vi "TCPIP_AcquisitionChA.vi"() -> ()   [LabVIEW 2018]
panel:
  out "error out 5":errorcluster
  out "error out":errorcluster
  in  "stop":bool
  out "error out 4":errorcluster
  out "error out 3":errorcluster
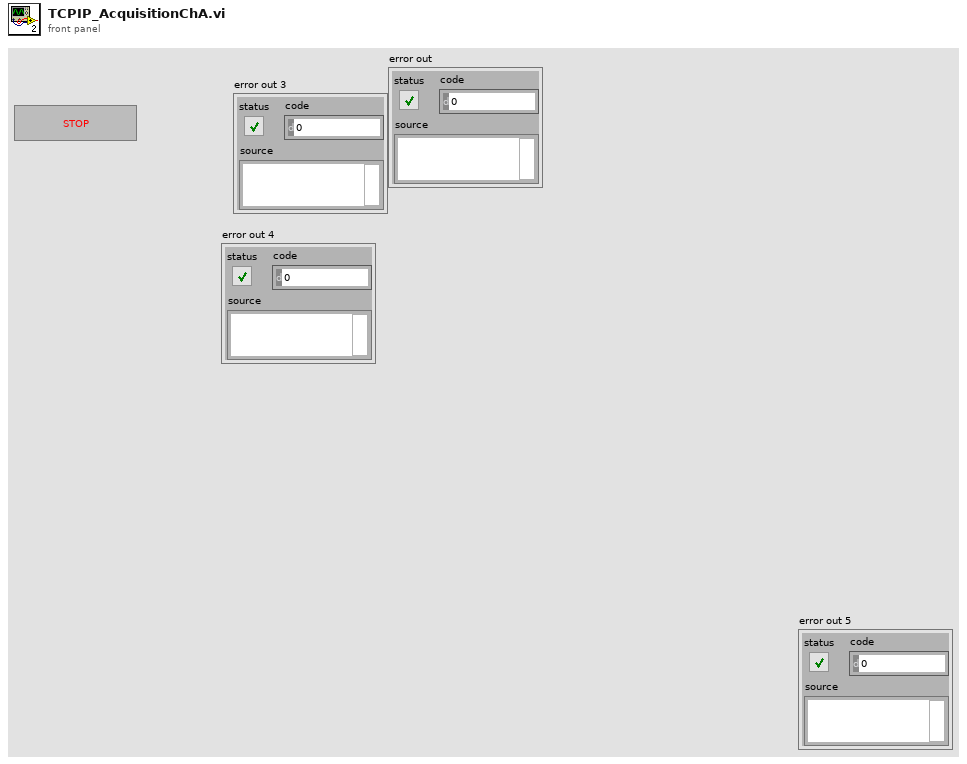
[diagram p1: front panel]
types:
  T1 = cluster{"ID":u32, "Address":string, "Service Name 1":string, "Service Name 2":string, "queue TX":refnum<queue>, "queue RX":refnum<queue>, "Port 1":u32, "Port 2":u32}
  T2 = enum16{"Standard", "Buffered", "CRLF", "Immediate"}
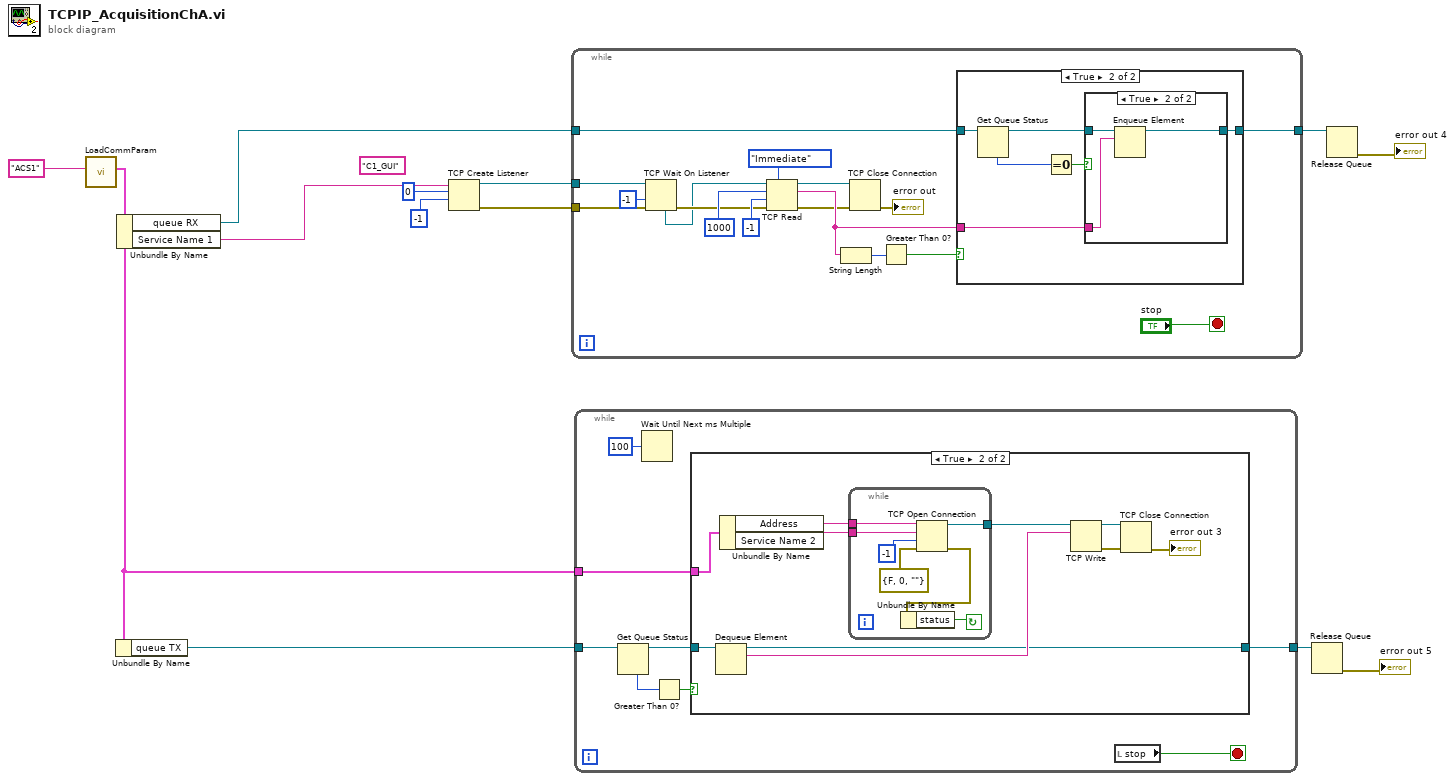
[diagram p0: block diagram]
diagram:
  (unwired) "C1_GUI" ("service name")
  n1 = call "LoadCommParam.vi"("section name"="ACS1") -> ("output cluster"=w2:T1)  [unwired: 10 in]
  n2 = Unbundle By Name(w2) -> ("queue TX"=w1:refnum<queue>)
  n3 = Unbundle By Name(w2) -> ("queue RX"=w4:refnum<queue>, "Service Name 1"=w3:string)
  n4 = TCP Create Listener(9:-1 ("timeout ms (25000)"), 10:u16 0 ("port"), 11:w3) -> (0:w10:errorcluster, 3:w11:refnum<k5>)  [unwired: 2 in, 1 out]
  n5 = while {
    tunnel: w4 -> [w29]
    tunnel: w11 -> [w22]
    tunnel: w10 -> [w19]
    tunnel: [w16] -> w9
    stop <- "stop" stop-if-true
    n6 = TCP Wait On Listener(8:w19, 9:-1 ("timeout ms (wait forever: -1)"), 11:w22) -> (0:w18:errorcluster, 4:w14:refnum<k5>)  [unwired: 1 in, 3 out]
    n7 = TCP Read(connection ID=w14, bytes to read=1000, error in (no error)=w18, 7:T2."Immediate" ("mode (standard)"), 9:-1 ("bytes to read")) -> (connection ID out=w21:refnum<k5>, data out=w26:string, error out=w20:errorcluster)
    n8 = String Length(string=w26) -> (length=w28:i32)
    n9 = TCP Close Connection(connection ID=w21, error in (no error)=w20) -> (error out=→"error out":errorcluster)  [unwired: 1 in, 1 out]
    n10 = Greater Than 0?(x=w28) -> (x > 0?=w27:bool)
    n11 = case shown="True" w27 {
      tunnel: w29 -> [w31 w35]
      tunnel: w26 -> [_ w33]
      tunnel: [w31 w32] -> w16
      frame False {
      }
      frame True {
        n12 = Get Queue Status(queue=w35) -> (queue out=w34:refnum<queue>, # elements in queue=w37:i32)  [unwired: 2 in, 6 out]
        n13 = Equal To 0?(x=w37) -> (x = 0?=w36:bool)
        n14 = case shown="True" w36 {
          tunnel: w34 -> [w38 w41]
          tunnel: w33 -> [_ w40]
          tunnel: [w38 w39] -> w32
          frame False {
          }
          frame True {
            n15 = Enqueue Element(queue=w41, element=w40) -> (queue out=w39:refnum<queue>)  [unwired: 2 in, 2 out]
          }
        }
      }
    }
  }
  n16 = while {
    tunnel: w1 -> [w49]
    tunnel: w2 -> [w45]
    tunnel: [w42] -> w6
    stop <- w43 stop-if-true
    n17 = Get Queue Status(queue=w49) -> (queue out=w46:refnum<queue>, # elements in queue=w48:i32)  [unwired: 2 in, 6 out]
    n18 = Wait Until Next ms Multiple(millisecond multiple=u32 100 ("milliseconds to wait")) -> ()  [unwired: 1 out]
    n19 = Greater Than 0?(x=w48) -> (x > 0?=w47:bool)
    n20 = case shown="True" w47 {
      tunnel: w46 -> [w50 w60]
      tunnel: w45 -> [_ w58]
      tunnel: [w50 w54] -> w42
      frame False {
      }
      frame True {
        n21 = Dequeue Element(queue=w60) -> (queue out=w54:refnum<queue>, element=w59:string)  [unwired: 2 in, 2 out]
        n22 = Unbundle By Name(w58) -> ("Address"=w56:string, "Service Name 2"=w55:string)
        n23 = while {
          tunnel: [w67] -> w57
          tunnel: w56 -> [w66]
          tunnel: w55 -> [w61]
          stop <- w62 continue-if-true
          n24 = TCP Open Connection(address=w66, remote port or service name=w61, timeout ms (60000)=-1, error in (no error)=errorcluster {"status"=FALSE, "code"=0, "source"=""}) -> (connection ID=w67:refnum<k5>, error out=w63:errorcluster)  [unwired: 1 in]
          n25 = Unbundle By Name(w63) -> ("status"=w62:bool)
        }
        n26 = TCP Write(connection ID=w57, data in=w59) -> (connection ID out=w51:refnum<k5>, error out=w53:errorcluster)  [unwired: 2 in, 1 out]
        n27 = TCP Close Connection(connection ID=w51, error in (no error)=w53) -> (error out=→"error out 3":errorcluster)  [unwired: 1 in, 1 out]
      }
    }
    n28 = local read "stop"() -> (w43:bool)
  }
  n29 = Release Queue(queue=w6) -> (error out=→"error out 5":errorcluster)  [unwired: 2 in, 2 out]
  n30 = Release Queue(queue=w9) -> (error out=→"error out 4":errorcluster)  [unwired: 2 in, 2 out]
